vi "CJCInitialise.vi"() -> (3 "Init Data Out":sgl[](array[numeric])=[-0.006458, 0.0059424504, 0.004802006, 0.0041854833, 0.003767837, 0.0034536726, 0.003203306, 0.002994881, 0.002817333, 0.00266208, 0.0025241822, 0.002400726, 0.0022885096, 0.0021854853, 0.0020908162, 0.0020024306, 0.0019198185, 0.0018421086, 0.0017691752, 0.001700014, 0.0016341978, 0.0015713646, 0.001511205, 0.0014534517, 0.0013978734, 0.0013447978, 0.0012934566, 0.0012432829, 0.0011948114, 0.0011483029, 0.0011022596, 0.0010579516, 0.001014559, 0.00097241614, 0.00093080243, 0.0008904312, 0.0008504058, 0.0008114728, 0.00077348645, 0.0007360942, 0.00069878076, 0.00066190877, 0.0006260307, 0.0005905767, 0.0005555098, 0.0005207951, 0.0004863991, 0.00045228965, 0.00041843578, 0.0003848077, 0.00035137613, 0.00031811287, 0.00028498995, 0.0002526055, 0.0002200558, 0.00018719044, 0.00015444802, 0.00012243993, 8.9676774e-05, 5.6775025e-05, 2.4174782e-05, -8.086018e-06, -4.0518757e-05, -7.391248e-05, -0.00010679401, -0.00013977663, -0.0001734326, -0.00020756602, -0.0002414478, -0.00027570827, -0.0003103916, -0.00034554527, -0.00038122086, -0.00041747428, -0.00045436702, -0.00049140316, -0.0005293472, -0.0005685925, -0.0006082109, -0.00064906076, -0.0006907765, -0.00073341856, -0.0007784969, -0.00082418876, -0.0008717023, -0.00092128344, -0.0009732275, -0.0010273166, -0.0010847201, -0.0011455452, -0.0012107727, -0.0012802035, -0.001357046, -0.0014403336, -0.0015344552, -0.0016420854, -0.0017685484, -0.0019250627, -0.0021359557, -0.0024757148])   [LabVIEW 2016]
panel:
  in  "Lookup Table":sgl[](array[numeric])=[-0.006458, 0.0059424504, 0.004802006, 0.0041854833, 0.003767837, 0.0034536726, 0.003203306, 0.002994881, 0.002817333, 0.00266208, 0.0025241822, 0.002400726, 0.0022885096, 0.0021854853, 0.0020908162, 0.0020024306, 0.0019198185, 0.0018421086, 0.0017691752, 0.001700014, 0.0016341978, 0.0015713646, 0.001511205, 0.0014534517, 0.0013978734, 0.0013447978, 0.0012934566, 0.0012432829, 0.0011948114, 0.0011483029, 0.0011022596, 0.0010579516, 0.001014559, 0.00097241614, 0.00093080243, 0.0008904312, 0.0008504058, 0.0008114728, 0.00077348645, 0.0007360942, 0.00069878076, 0.00066190877, 0.0006260307, 0.0005905767, 0.0005555098, 0.0005207951, 0.0004863991, 0.00045228965, 0.00041843578, 0.0003848077, 0.00035137613, 0.00031811287, 0.00028498995, 0.0002526055, 0.0002200558, 0.00018719044, 0.00015444802, 0.00012243993, 8.9676774e-05, 5.6775025e-05, 2.4174782e-05, -8.086018e-06, -4.0518757e-05, -7.391248e-05, -0.00010679401, -0.00013977663, -0.0001734326, -0.00020756602, -0.0002414478, -0.00027570827, -0.0003103916, -0.00034554527, -0.00038122086, -0.00041747428, -0.00045436702, -0.00049140316, -0.0005293472, -0.0005685925, -0.0006082109, -0.00064906076, -0.0006907765, -0.00073341856, -0.0007784969, -0.00082418876, -0.0008717023, -0.00092128344, -0.0009732275, -0.0010273166, -0.0010847201, -0.0011455452, -0.0012107727, -0.0012802035, -0.001357046, -0.0014403336, -0.0015344552, -0.0016420854, -0.0017685484, -0.0019250627, -0.0021359557, -0.0024757148]
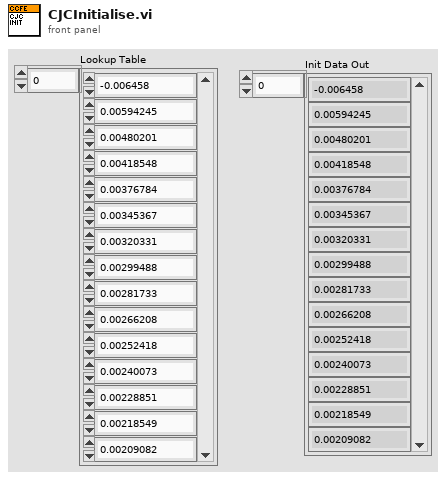
[diagram p1: front panel]
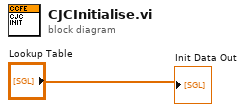
[diagram p0: block diagram]
diagram:
  "Init Data Out" <- "Lookup Table"
